vi "Com_Matrix220_String To Bitmap.vi"(3 "String":string) -> (0 "Image Data":T1, 1 "Error Tips":T2)   [LabVIEW 2016]
uses:
  <vilib>/picture/picture.llb/imagedata.ctl
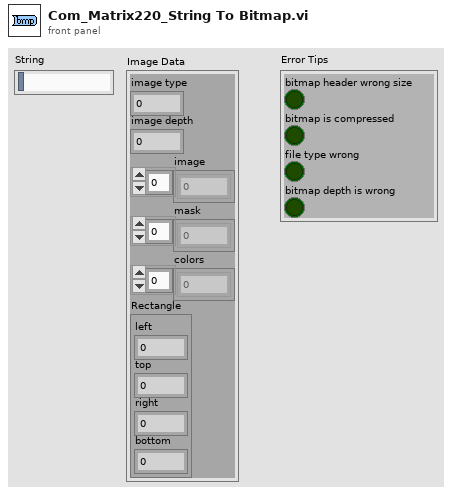
[diagram p1: front panel]
types:
  T1 = typedef "imagedata.ctl" = cluster{"image type":i32, "image depth":i32, "image":u8[], "mask":u8[], "colors":u32[], "Rectangle":cluster{"left":i16, "top":i16, "right":i16, "bottom":i16}}
  T2 = cluster{"bitmap header wrong size":bool, "bitmap is compressed":bool, "file type wrong":bool, "bitmap depth is wrong":bool}
  T3 = cluster{"left":i16, "top":i16, "right":i16, "bottom":i16}
  T4 = cluster{"height":u32, "width":u32, "bit depth":u16, "padded width":u32}
  T5 = cluster{"[0]":bool, "[1]":bool, "[2]":bool, "[3]":bool}
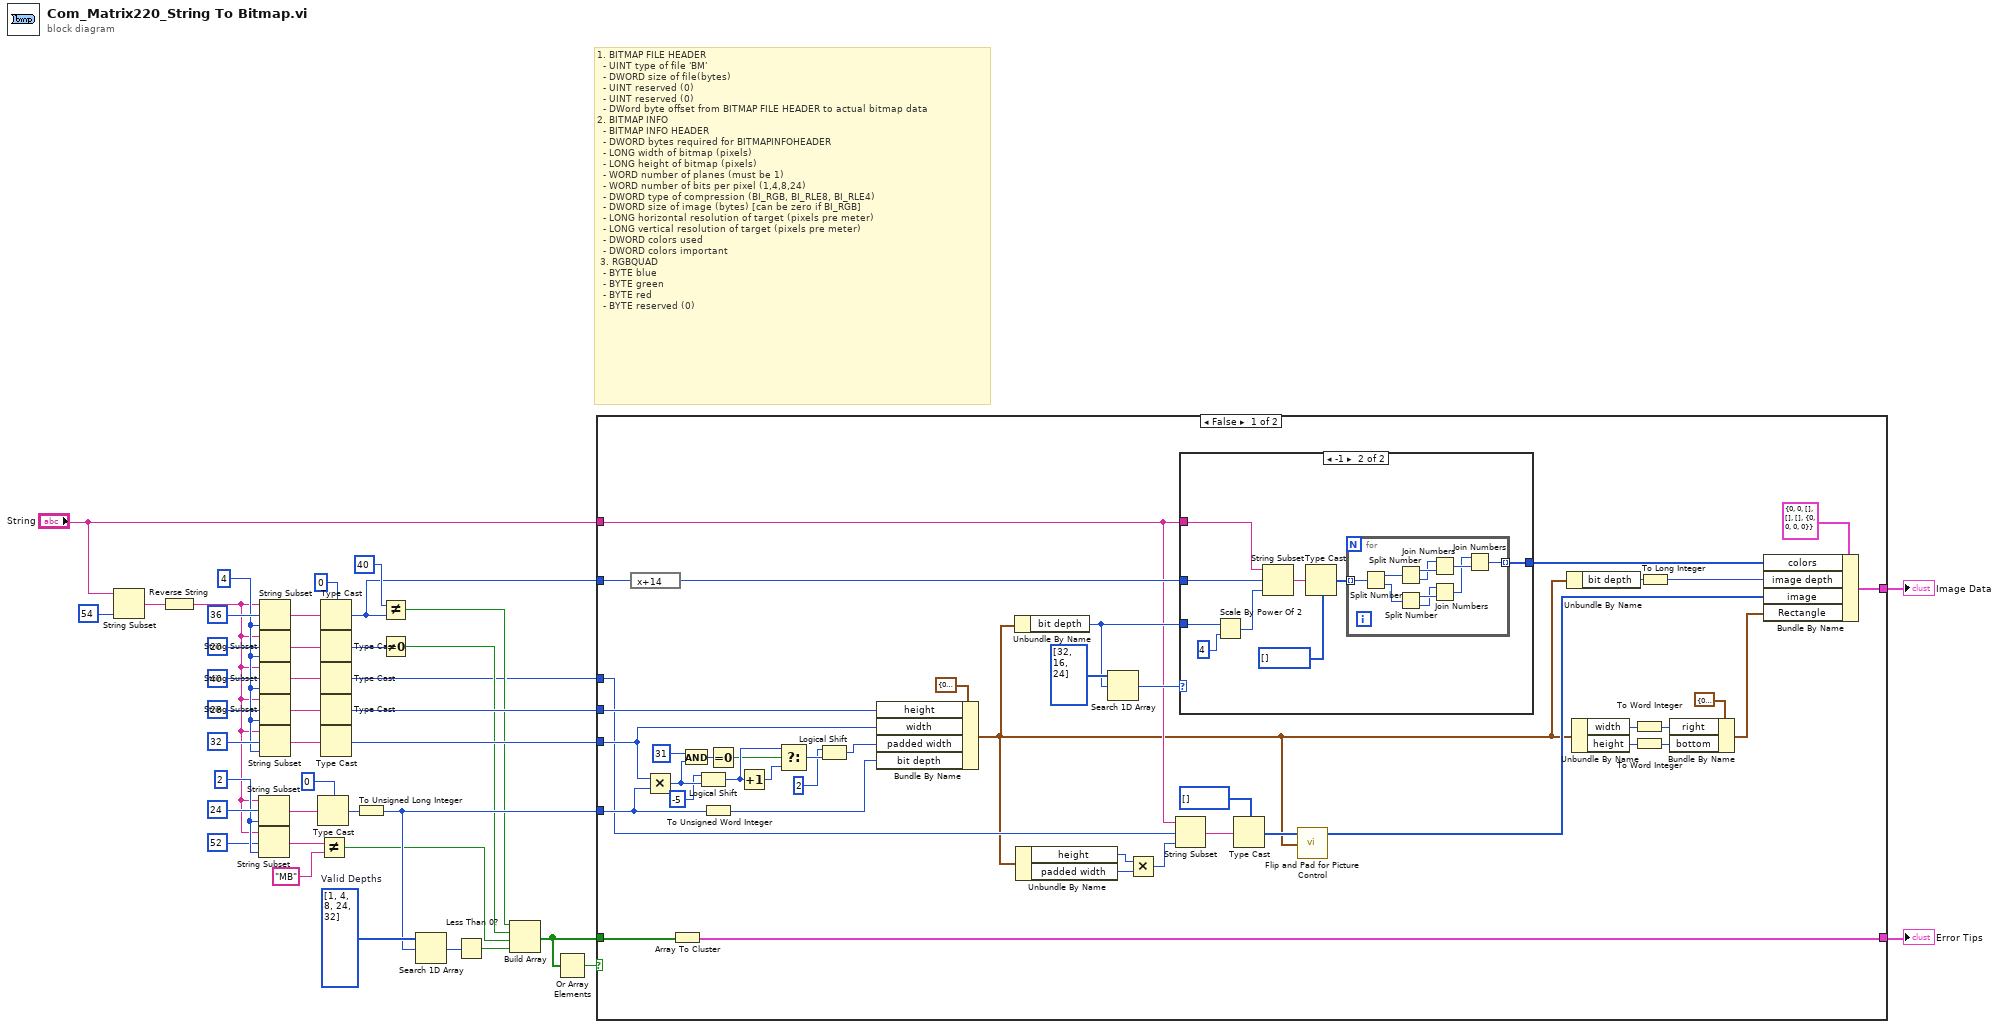
[diagram p0: block diagram]
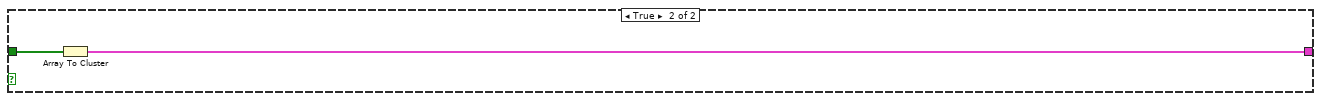
[diagram p3: hidden frame]
diagram:
  w14 = u32[] [1, 4, 8, 24, 32]  # Valid Depths
  w31 = 2 ("length (rest)")
  w22 = u32 0
  w32 = 4 ("length (rest)")
  # "1. BITMAP FILE HEADER\n  - UINT\ttype of file 'BM'\n  - DWORD\tsize of file(bytes)\n  - UINT\treserved (0)\n  - UINT\treserved (0)\n  - DWord\tbyte offset from BITMAP FILE HEADER to actual bitmap data\n2. BITMAP INFO\n  - BITMAP INFO HEADER\n  - DWORD\tbytes required for BITMAPINFOHEADER\n  - LONG\twidth of bitmap (pixels)\n  - LONG\theight of bitmap (pixels)\n  - WORD\tnumber of planes (must be 1)\n  - WORD\tnumber of bits per pixel (1,4,8,24)\n  - DWORD\ttype of compression (BI_RGB, BI_RLE8, BI_RLE4)\n  - DWORD\tsize of image (bytes) [can be zero if BI_RGB]\n  - LONG\thorizontal resolution of target (pixels pre meter)\n  - LONG\tvertical resolution of target (pixels pre meter)\n  - DWORD\tcolors used\n  - DWORD\tcolors important\n 3. RGBQUAD\n  - BYTE\tblue\n  - BYTE\tgreen\n  - BYTE\tred\n  - BYTE\treserved (0)"
  n1 = String Subset(string="String", length (rest)=54 ("length (rest)")) -> (substring=w40:string)  [unwired: 1 in]
  n2 = Reverse String(1:w40) -> (0:w30:string)
  n3 = String Subset(string=w30, offset (0)=24, length (rest)=w31) -> (substring=w21:string)
  n4 = String Subset(string=w30, offset (0)=52, length (rest)=w31) -> (substring=w19:string)
  n5 = String Subset(string=w30, offset (0)=36, length (rest)=w32) -> (substring=w38:string)
  n6 = String Subset(string=w30, offset (0)=20, length (rest)=w32) -> (substring=w27:string)
  n7 = String Subset(string=w30, offset (0)=40, length (rest)=w32) -> (substring=w25:string)
  n8 = String Subset(string=w30, offset (0)=28, length (rest)=w32) -> (substring=w24:string)
  n9 = String Subset(string=w30, offset (0)=32, length (rest)=w32) -> (substring=w23:string)
  n10 = Type Cast(type=u16 0, x=w21) -> (*(type *) &x=w17:u16)
  n11 = Not Equal?(x=w19, y="MB") -> (x != y?=w9:bool)
  n12 = Type Cast(type=w22, x=w38) -> (*(type *) &x=w5:u32)
  n13 = Type Cast(type=w22, x=w27) -> (*(type *) &x=w26:u32)
  n14 = Type Cast(type=w22, x=w25) -> (*(type *) &x=w3:u32)
  n15 = Type Cast(type=w22, x=w24) -> (*(type *) &x=w16:u32)
  n16 = Type Cast(type=w22, x=w23) -> (*(type *) &x=w15:u32)
  n17 = To Unsigned Long Integer(number=w17) -> (unsigned 32bit integer=w13:u32)
  n18 = Not Equal?(x=u32 40, y=w5) -> (x != y?=w11:bool)
  n19 = Not Equal To 0?(x=w26) -> (x != 0?=w10:bool)
  n20 = Search 1D Array(1D array=w14, element=w13) -> (index of element=w12:i32)  [unwired: 1 in]
  n21 = Less Than 0?(x=w12) -> (x < 0?=w8:bool)
  n22 = Build Array(w11, w10, w9, w8) -> (w6:bool[])
  n23 = Or Array Elements(Boolean array=w6) -> (logical OR=w7:bool)
  n24 = case shown="False" w7 {
    tunnel: w16 -> [w74 _]
    tunnel: w15 -> [w73 _]
    tunnel: w13 -> [w70 _]
    tunnel: w6 -> [w43 w105]
    tunnel: w5 -> [w69 _]
    tunnel: "String" -> [w59 _]
    tunnel: w3 -> [w58 _]
    tunnel: [w44 _] -> w2
    tunnel: [w42 w104] -> w1
    frame False {
      n25 = expression code="x+14"(w69) -> (w66:u32)
      n26 = Multiply(x=w73, y=w70) -> (x*y=w77:u32)
      n27 = Array To Cluster(array=w43) -> (cluster=w42:T5)
      n28 = And(x=u32 31, y=w77) -> (x .and. y?=w79:u32)
      n29 = Logical Shift(y=-5, x=w77) -> (x << y=w81:u32)
      n30 = To Unsigned Word Integer(number=w70) -> (unsigned 16bit integer=w71:u16)
      n31 = Equal To 0?(x=w79) -> (x = 0?=w80:bool)
      n32 = Increment(x=w81) -> (x+1=w82:u32)
      n33 = Select(t=w81, s=w80, f=w82) -> (s? t:f=w84:u32)
      n34 = Logical Shift(y=2, x=w84) -> (x << y=w72:u32)
      n35 = Bundle By Name(cluster=T4 {"height"=0, "width"=0, "bit depth"=0, "padded width"=0} ("bitmap info"), "height"=w74, "width"=w73, "padded width"=w72, "bit depth"=w71) -> (w50:T4)
      n36 = Unbundle By Name(w50) -> ("bit depth"=w65:u16)
      n37 = Unbundle By Name(w50) -> ("height"=w60:u32, "padded width"=w61:u32)
      n38 = Search 1D Array(1D array=u16[] [32, 16, 24], element=w65) -> (index of element=w67:i32)  [unwired: 1 in]
      n39 = Multiply(x=w60, y=w61) -> (x*y=w57:u32)
      n40 = String Subset(string=w59, offset (0)=w58, length (rest)=w57) -> (substring=w56:string)
      n41 = case shown="-1" w67 {
        tunnel: w59 -> [_ w93]
        tunnel: w66 -> [_ w92]
        tunnel: w65 -> [_ w91]
        tunnel: [_ w85] -> w52
        frame Default {
        }
        frame -1 {
          n42 = Scale By Power Of 2(n=w91, x=4) -> (x*2^n=w89:i32)
          n43 = String Subset(string=w93, offset (0)=w92, length (rest)=w89) -> (substring=w88:string)
          n44 = Type Cast(type=u32[] [], x=w88) -> (*(type *) &x=w86:u32[])
          n45 = for {
            tunnel: w86 -> [w103] mode=indexing
            tunnel: [w94] -> w85 mode=indexing
            n46 = Split Number(x=w103) -> (hi(x)=w102:u16, lo(x)=w101:u16)
            n47 = Split Number(x=w102) -> (hi(x)=w100:u8, lo(x)=w99:u8)
            n48 = Split Number(x=w101) -> (hi(x)=w98:u8, lo(x)=w97:u8)
            n49 = Join Numbers(hi=w99, lo=w100) -> ((hi.lo)=w96:u16)
            n50 = Join Numbers(hi=w97, lo=w98) -> ((hi.lo)=w95:u16)
            n51 = Join Numbers(hi=w95, lo=w96) -> ((hi.lo)=w94:u32)
          }
        }
      }
      n52 = Type Cast(type=u8[] [], x=w56) -> (*(type *) &x=w54:u8[])
      n53 = call <vilib>:"Flip and Pad for Picture Control.vi"("bitmap info"=w50, "BMP bitmap"=w54) -> ("picture bitmap"=w53:u8[])  [unwired: 3 in]
      n54 = Unbundle By Name(w50) -> ("bit depth"=w63:u16)
      n55 = Unbundle By Name(w50) -> ("width"=w49:u32, "height"=w47:u32)
      n56 = To Word Integer(number=w49) -> (16bit integer=w48:i16)
      n57 = To Word Integer(number=w47) -> (16bit integer=w46:i16)
      n58 = To Long Integer(number=w63) -> (32bit integer=w62:i32)
      n59 = Bundle By Name(cluster=T3 {"left"=0, "top"=0, "right"=0, "bottom"=0} ("Rectangle"), "right"=w48, "bottom"=w46) -> (w45:T3)
      n60 = Bundle By Name(cluster=T1 {"image type"=0, "image depth"=0, "image"=[], "mask"=[], "colors"=[], "Rectangle"={"left"=0, "top"=0, "right"=0, "bottom"=0}} ("image data"), "colors"=w52, "image depth"=w62, "image"=w53, "Rectangle"=w45) -> (w44:T1)
    }
    frame True {
      n61 = Array To Cluster(array=w105) -> (cluster=w104:T5)
    }
  }
  "Error Tips" <- w1
  "Image Data" <- w2
